vi "Get Module Identifier.vi"(8 "error in":errorcluster, 10 "module path":string, 11 "routing and faulting in":T1 format="%.0x") -> (0 "error out":errorcluster, 1 "found?":bool, 2 "module identifier":string, 3 "routing and faulting out":T1 format="%.0x")   [LabVIEW 2020, in "Routing and Faulting Scripting.lvlib"]
uses:
  Routing and Faulting Scripting.lvlib
  <vilib>/NI VeriStand/Custom Device API/Custom Device Item Ref.ctl
  NationalInstruments.VeriStand.SystemStorage
  <vilib>/NI VeriStand/Custom Device API/Custom Device API.lvlib
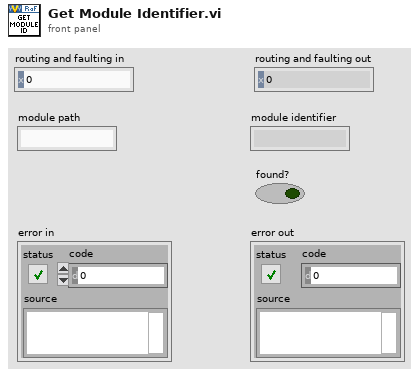
[diagram p1: front panel]
types:
  T1 = typedef "Custom Device API.lvlib/Custom Device Item Ref.ctl" = u64
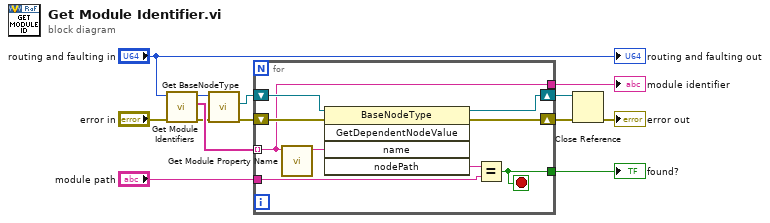
[diagram p0: block diagram]
diagram:
  n1 = call "Get Module Identifiers.vi"("error in"="error in", "routing and faulting in"="routing and faulting in") -> ("error out"=w3:errorcluster, "module Identifier"=w12:string[], "routing and faulting out"=w1:T1)  [unwired: 7 in]
  n2 = call "Get BaseNodeType.vi"("error in"=w3, "item in"=w1) -> ("error out"=w2:errorcluster, "BaseNodeType"=w4:refnum<k24>)  [unwired: 7 in, 1 out]
  n3 = for {
    tunnel: w12 -> [w14] mode=indexing
    tunnel: "module path" -> [w15]
    tunnel: [w14] -> w13
    shift-right: [w19] -> w10
    shift-left: w2 -> [w22]
    tunnel: [w18] -> w9
    shift-right: [w17] -> w7
    shift-left: w4 -> [w21]
    stop <- w18 stop-if-true
    n4 = call "Get Module Property Name.vi"("module identifier"=w14) -> ("module property name"=w16:string)  [unwired: 10 in]
    n5 = invoke class="BaseNodeType" method="GetDependentNodeValue"(reference=w21, error in=w22, "name"=w16) -> (reference out=w17:refnum<k24>, error out=w19:errorcluster, "nodePath"=w20:string)  [unwired: 2 in, 2 out]
    n6 = Equal?(x=w20, y=w15) -> (x = y?=w18:bool)
  }
  "module identifier" <- w13
  "found?" <- w9
  n7 = Close Reference(reference=w7, error in (no error)=w10) -> (error out=→"error out":errorcluster)
  "routing and faulting out" <- "routing and faulting in"
